vi "参数设置页.vi"() -> ()   [LabVIEW 2016, in "挥发酚.lvlib"]
uses:
  <vilib>/Plasmionique/MB Master/MB_Master/MB_Master.lvclass
  <vilib>/ptbypt/NI_PtbyPt.lvlib
panel:
  in  "维护模式":bool
  in  "标样核查自动补测":bool caption="通讯连接"
  in  "跨度核查自动补测":bool caption="通讯连接"
  in  "零点核查自动补测":bool caption="通讯连接"
  in  "标样核查标液偏差":dbl caption="标样核查标液偏差："
  in  "跨度核查标液偏差":dbl caption="跨度核查标液偏差："
  in  "零点核查标液偏差":dbl caption="零点核查标液偏差："
  out "error out":errorcluster
  out "数据刷新时间":string
  in  "通讯连接":bool
  out "MB table":enum32{"Serial", "TCP"}(tab)
  in  "请选择串口:":refnum<visa-resource-name>
  in  "IP":string="127.0.0.1"
  in  "PORT":string="1001"
  in  "通信方式选择":enum16{"串口", "TCP"}(ring)
  in  "刷新":bool
  in  "参数下拉列表":u16(ring)=1 items=["挥发酚"=1]
  in  "量程下拉列表":enum16{"低量程", "高量程"}(ring)
  out "量程下限":dbl caption="量程下限："
  out "量程上限":dbl caption="量程上限："
  out "检出限":dbl caption="检出限："
  out "曲线截距":dbl caption="曲线截距：" format="%#.6f"
  out "曲线斜率":dbl caption="曲线斜率：" format="%#.6f"
  out "二次多项式系数":dbl caption="二次多项式系数：" format="%#.6f"
  out "消解时长":dbl caption="消解时长："
  out "消解温度":dbl caption="消解温度："
  out "测量精度":dbl caption="测量精度："
  in  "标样核查标液浓度":dbl caption="标样核查标液浓度："
  in  "跨度核查标液浓度":dbl caption="跨度核查标液浓度："
  in  "零点核查标液浓度":dbl caption="零点核查标液浓度："
  in  "跨度值":dbl caption="跨度值："
  # "日质控设置"
  # "日质控自动补测设置"
  # "连接设置"
  # "±"
  # "%"
  # "%"
  # "关键参数"
  # "线性公式"
  # "mg/L"
  # "mg/L"
  # "mg/L"
  # "℃"
  # "min"
  # "mg/L"
  # "mg/L"
  # "mg/L"
  # "mg/L"
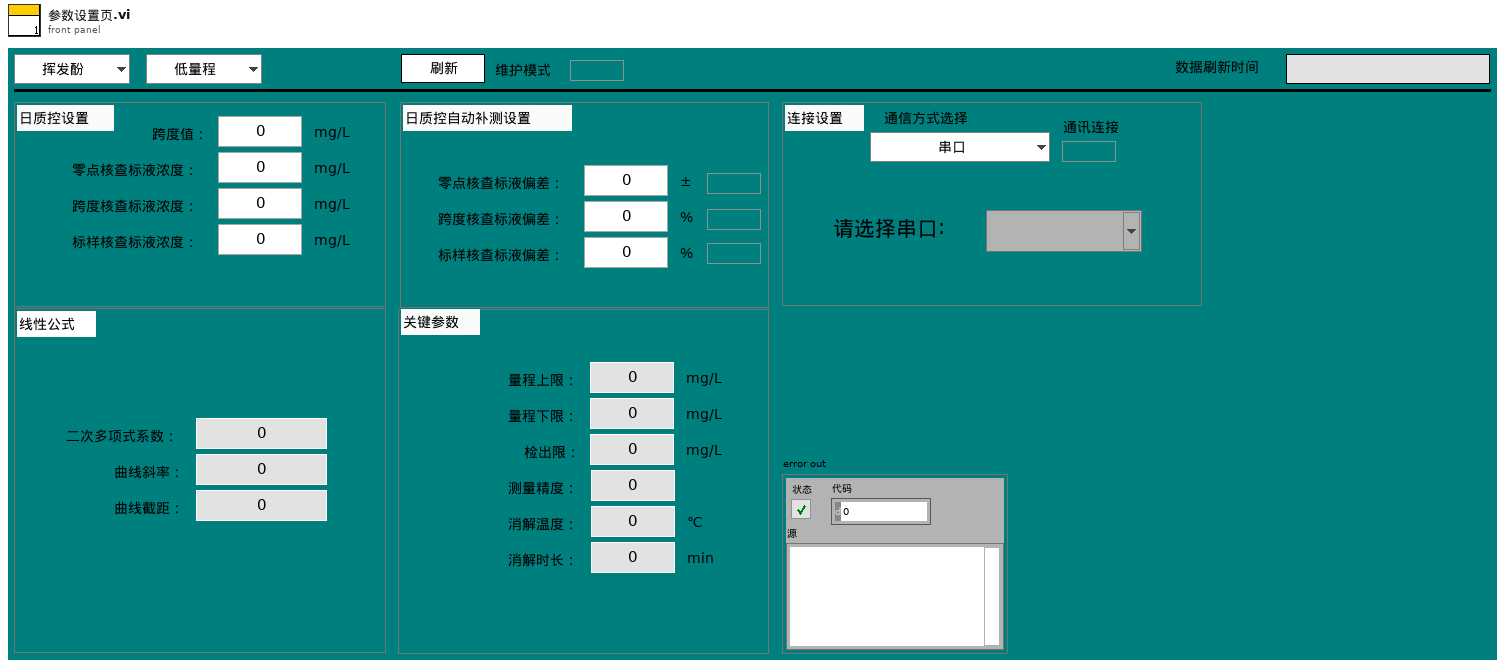
[diagram p1: front panel]
types:
  T1 = enum8{"Enabled", "Disabled", "Disabled and Grayed Out"}
  T2 = cluster{"跨度值":dbl, "零点标准液浓度":dbl, "跨度标准液浓度":dbl, "标准液标准浓度":dbl, "零点标准液偏差":dbl, "跨度标准液偏差":dbl, "标准液标准偏差":dbl}
  T3 = cluster{"测量量程":sgl, "测量检出限":sgl, "测量精度":sgl, "测量间隔":sgl, "消解温度":sgl, "消解时长":sgl, "三项式系数":sgl, "二次多项式系数":sgl, "曲线斜率":sgl, "曲线截距":sgl, "线性相关系数":sgl, "空白校准时间":timestamp, "标样校准时间":timestamp, "测量信号值":sgl, "稀释倍数":sgl, "量程系数":sgl}
  T4 = cluster{"测量精度":u16, "消解温度":u16, "消解时长":u16, "量程下限":sgl, "量程上限":sgl, "曲线斜率K":sgl, "曲线斜率B":sgl, "标定日期":timestamp, "标液1浓度":sgl, "标液1测量过程值":sgl, "标液2浓度":sgl, "标液2测量过程值":sgl, "标液3浓度":sgl, "标液3测量过程值":sgl, "标液4浓度":sgl, "标液4测量过程值":sgl, "标液5浓度":sgl, "标液5测量过程值":sgl, "线性相关系数":sgl, "试剂余量":u32, "测量滴定值或吸光度":sgl, "标样2校准时间":timestamp, "检出限值":sgl, "校准系数":sgl, "设备系列号":string, "显色温度":u16, "显色时间":u16, "试剂余量1":u16, "试剂余量2":u16, "试剂余量3":u16, "试剂余量4":u16, "试剂余量5":u16, "试剂余量6":u16, "试剂余量7":u16, "试剂余量8":u16, "试剂余量9":u16, "试剂余量10":u16, "当前量程低位":sgl, "当前量程高位":sgl}
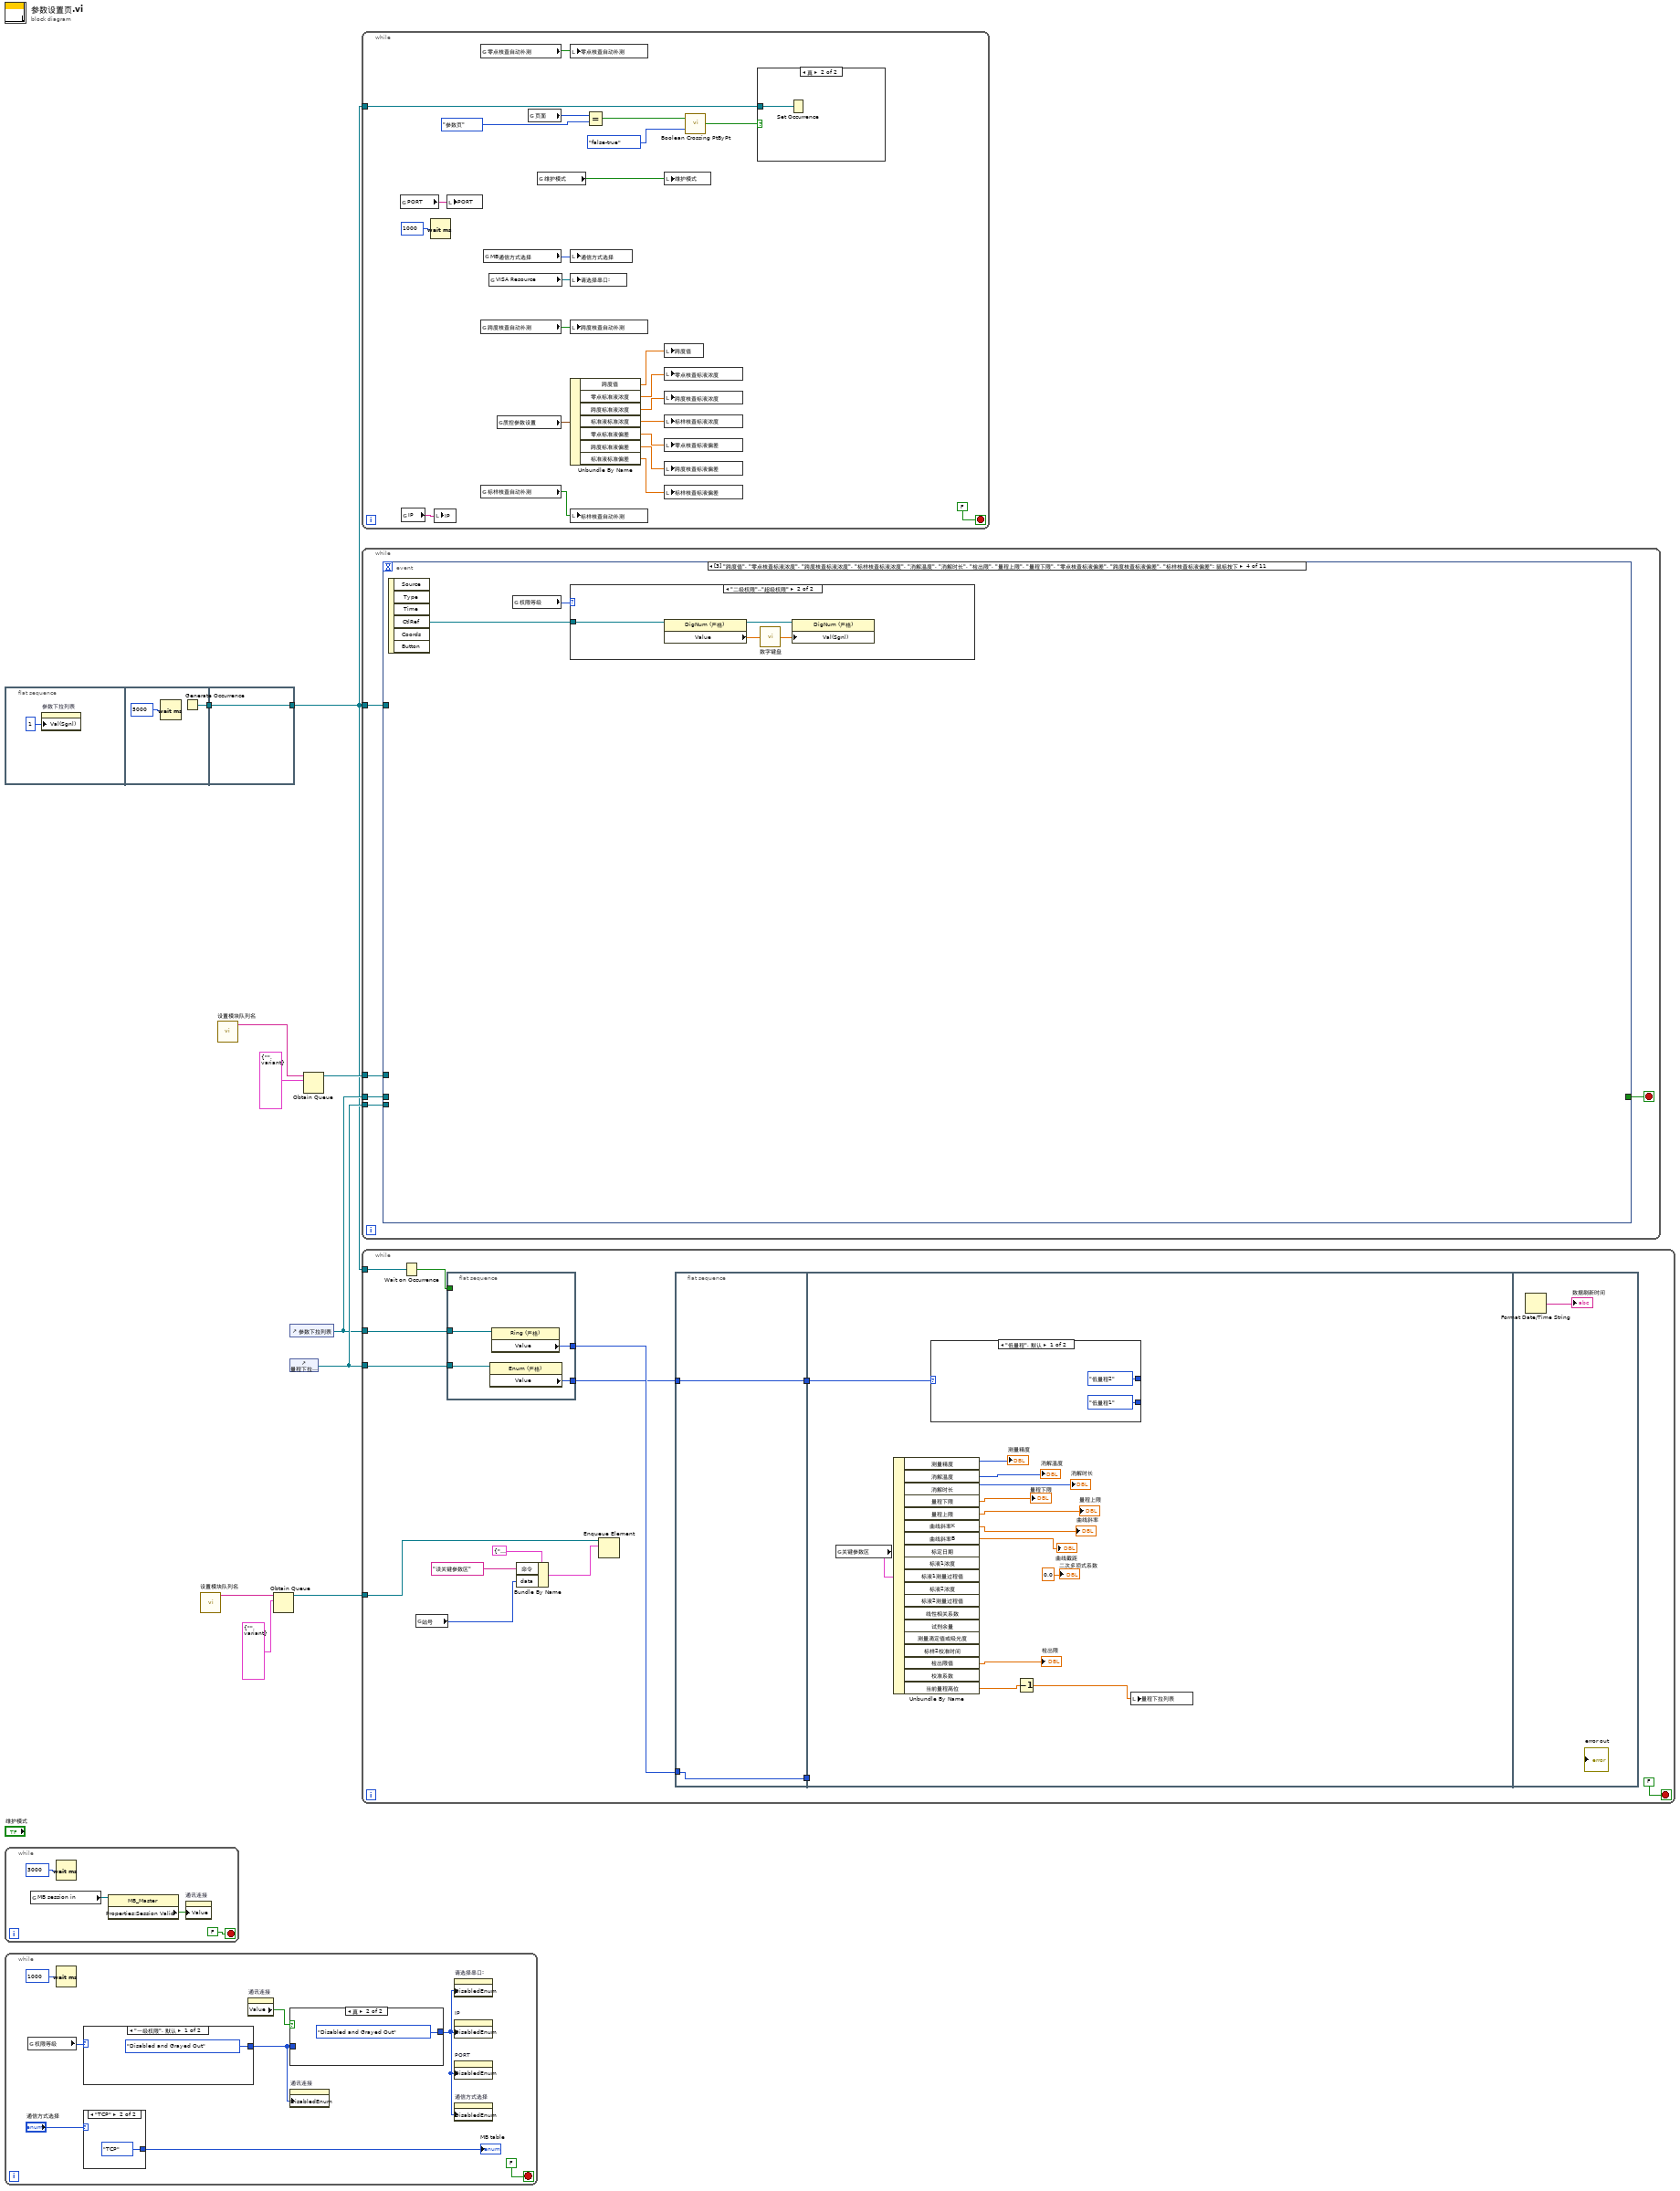
[diagram p0: block diagram]
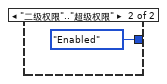
[diagram p3: hidden frame]
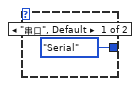
[diagram p4: hidden frame]
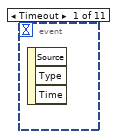
[diagram p6: hidden frame]
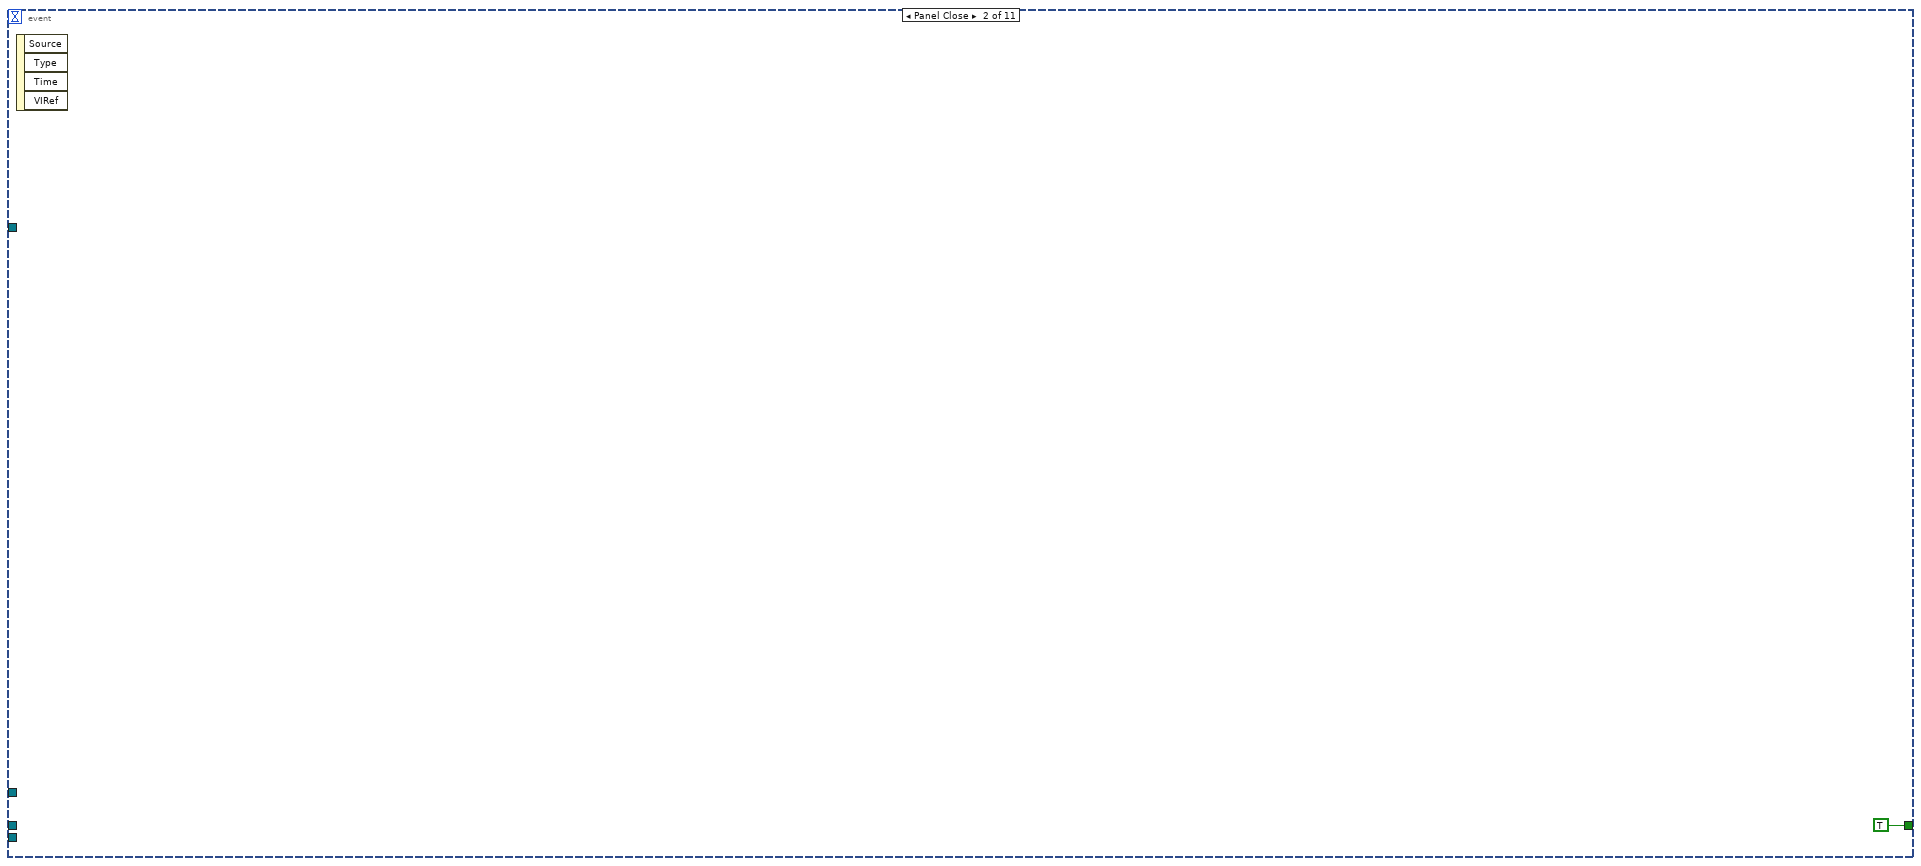
[diagram p7: hidden frame]
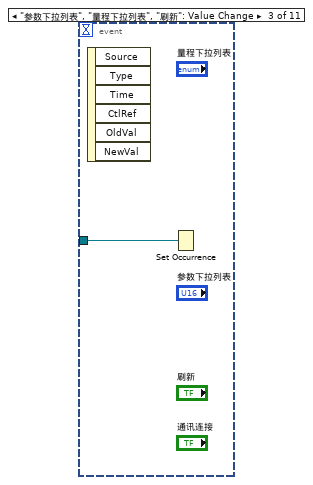
[diagram p8: hidden frame]
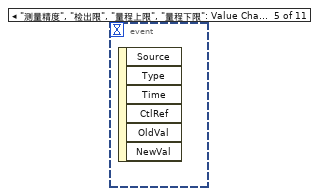
[diagram p10: hidden frame]
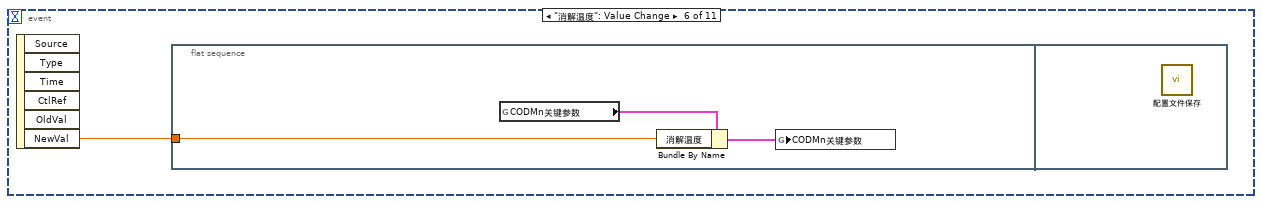
[diagram p11: hidden frame]
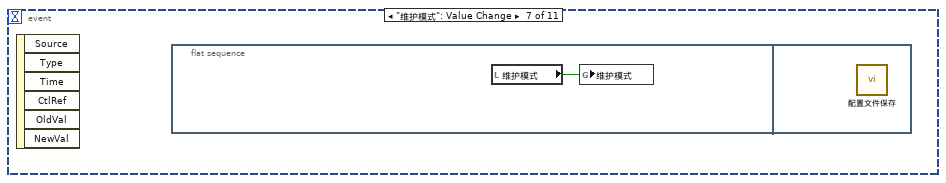
[diagram p12: hidden frame]
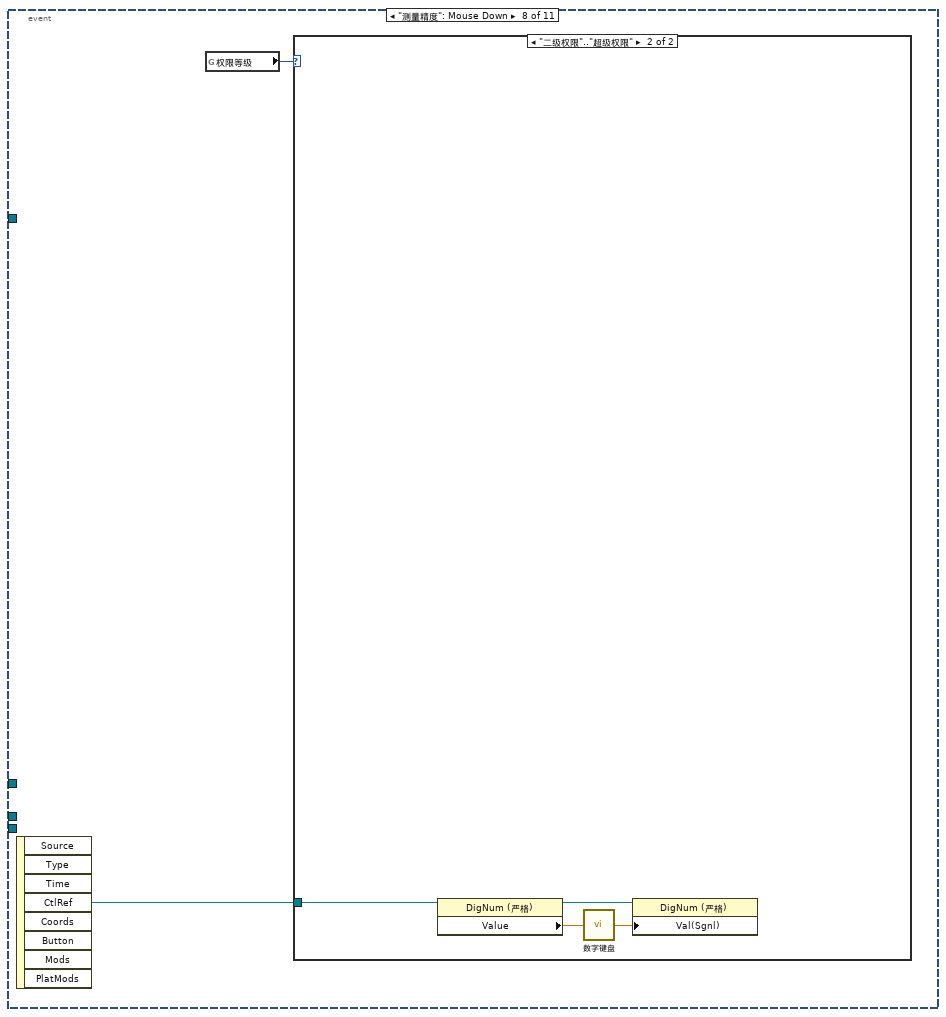
[diagram p13: hidden frame]
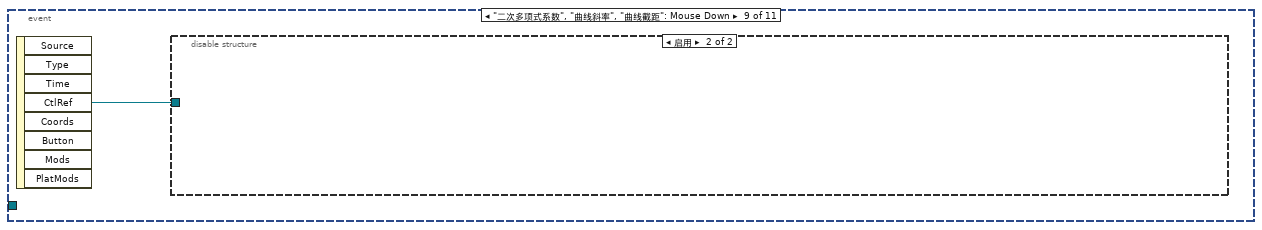
[diagram p15: hidden frame]
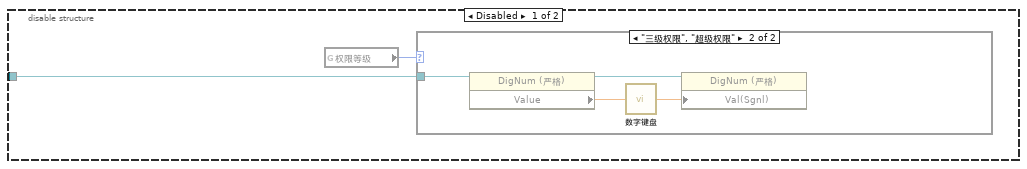
[diagram p16: hidden frame]
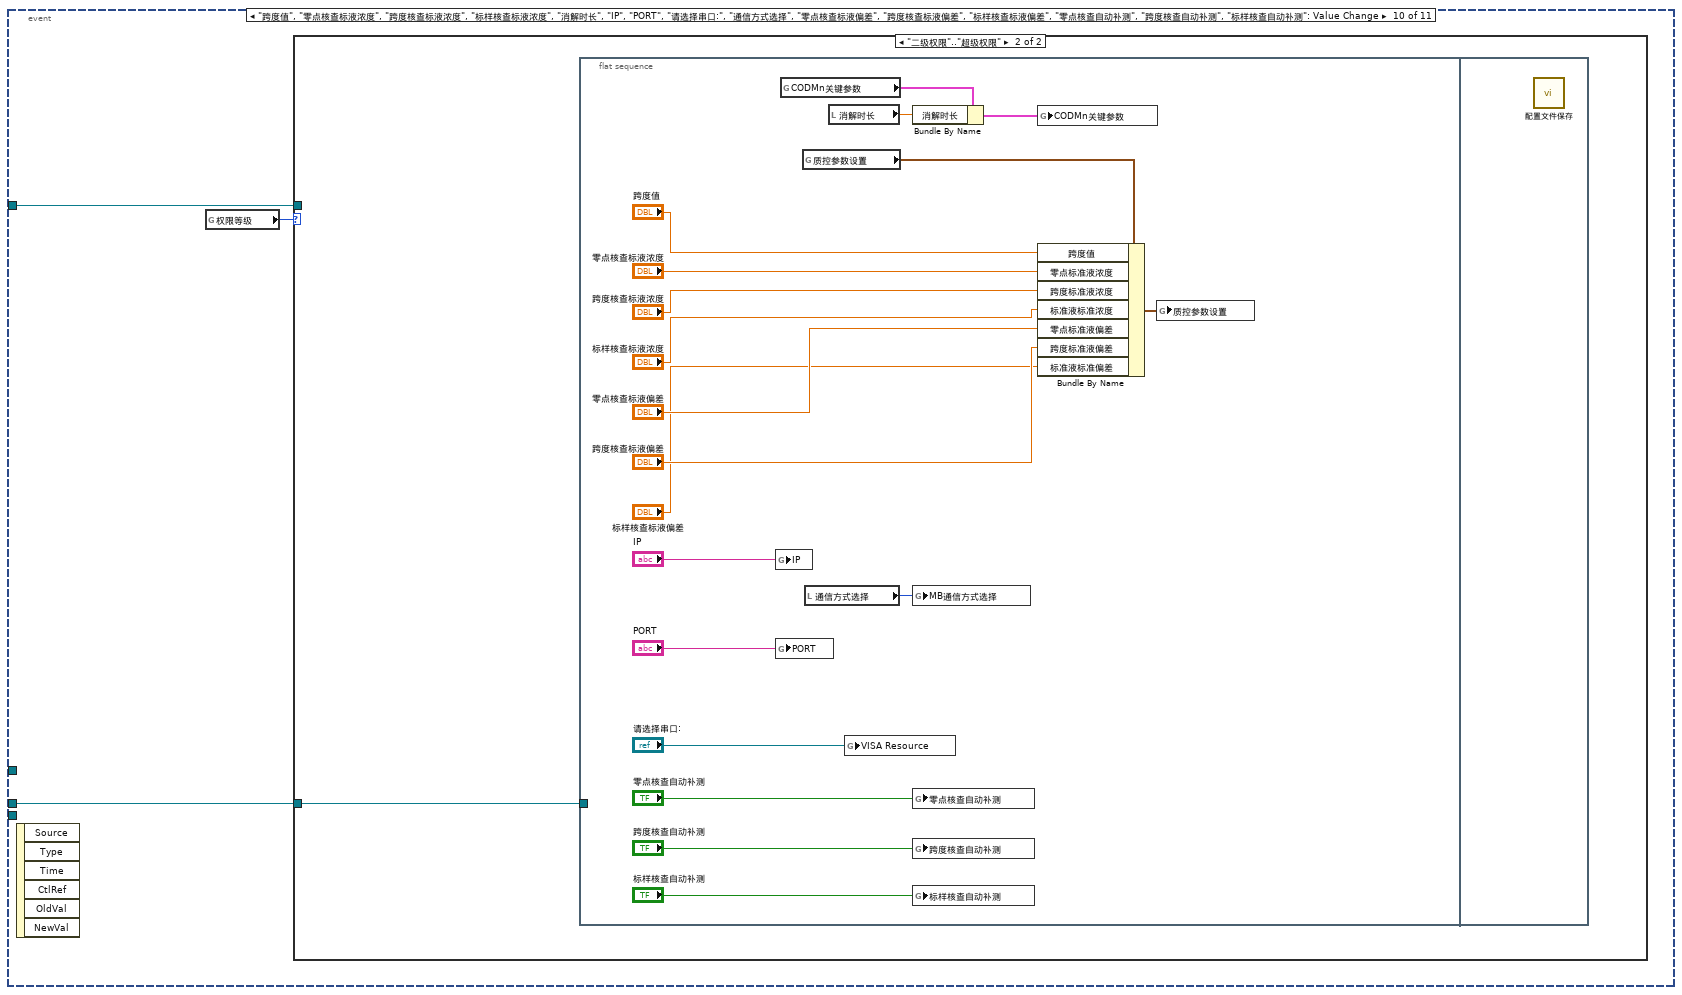
[diagram p18: hidden frame]
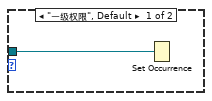
[diagram p19: hidden frame]
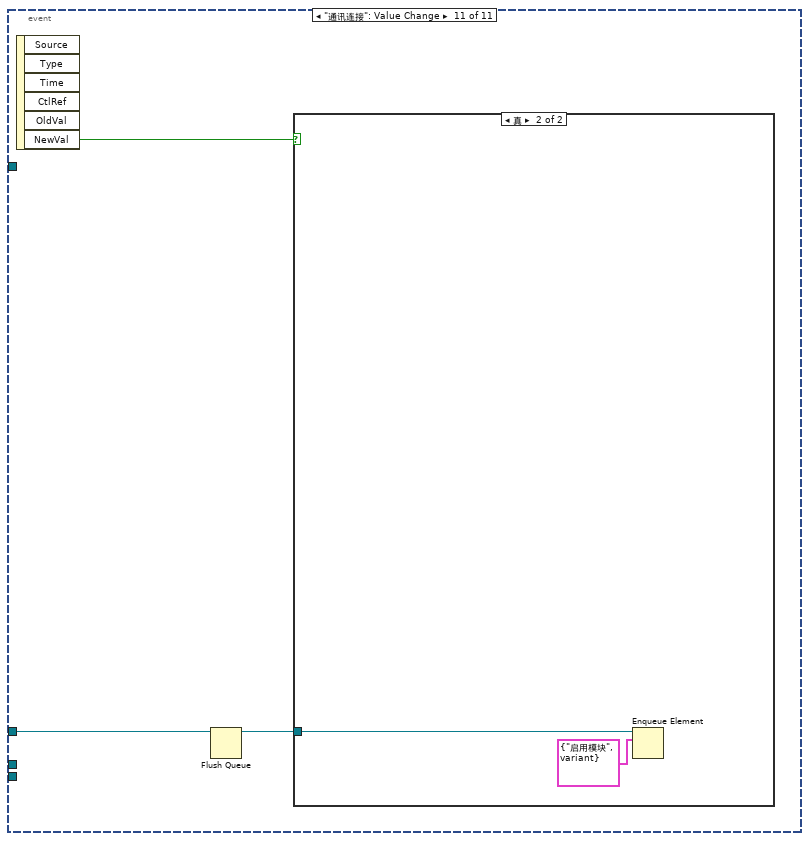
[diagram p20: hidden frame]
diagram:
  n1 = flat-sequence {
    tunnel: [w13] -> w10
    tunnel: [w14] -> w5
    tunnel: w10 -> [w14]
    frame #0 {
      n2 = property on="参数下拉列表" class="Ring (严格)"("Val(Sgnl)"=u16 1 ("值(信号)")) -> ()  [unwired: 2 in, 2 out]
    }
    frame #1 {
      n3 = Wait (ms)(milliseconds to wait=u32 5000 ("等待时间（毫秒）")) -> ()  [unwired: 1 out]
      n4 = Generate Occurrence() -> (w13:refnum<k4>)
    }
    frame #2 {
    }
  }
  n5 = while {
    stop <- FALSE stop-if-true
    n6 = global read "VAR挥发酚全局变量.vi" "MB session in"() -> (w17:refnum<class "MB_Master.lvclass">)
    n7 = Wait (ms)(milliseconds to wait=u32 3000 ("等待时间（毫秒）")) -> ()  [unwired: 1 out]
    n8 = property class="MB_Master"(reference=w17) -> ("Properties:Session Valid"=w16:bool)  [unwired: 1 in, 2 out]
    n9 = property on="通讯连接" class="Bool (严格)"("Value"=w16) -> ()  [unwired: 2 in, 2 out]
  }
  n10 = while {
    stop <- FALSE stop-if-true
    n11 = global read "VAR挥发酚全局变量.vi" "权限等级"() -> (w19:enum16{"一级权限", "二级权限", "三级权限", "超级权限"})
    n12 = Wait (ms)(milliseconds to wait=u32 1000 ("等待时间（毫秒）")) -> ()  [unwired: 1 out]
    n13 = case shown="\"一级权限\", 默认" w19 {
      tunnel: [T1."Disabled and Grayed Out" ("禁用") T1."Enabled" ("禁用")] -> w20
      frame "一级权限", Default {
      }
      frame "二级权限".."超级权限" {
      }
    }
    n14 = case shown="\"TCP\"" "通信方式选择" {
      tunnel: [enum32{"Serial", "TCP"}."Serial" ("MB table") enum32{"Serial", "TCP"}."TCP" ("MB table")] -> w22
      frame "串口", Default {
      }
      frame "TCP" {
      }
    }
    "MB table" <- w22
    n15 = property on="通讯连接" class="Bool (严格)"() -> ("Value"=w24:bool)  [unwired: 2 in, 2 out]
    n16 = case shown="真" w24 {
      tunnel: [w31 T1."Disabled and Grayed Out" ("禁用")] -> w23
      tunnel: w20 -> [w31 _]
      frame False {
      }
      frame True {
      }
    }
    n17 = property on="通讯连接" class="Bool (严格)"("DisabledEnum"=w20) -> ()  [unwired: 2 in, 2 out]
    n18 = property on="请选择串口:" class="VISAName"("DisabledEnum"=w23) -> ()  [unwired: 2 in, 2 out]
    n19 = property on="IP" class="Str"("DisabledEnum"=w23) -> ()  [unwired: 2 in, 2 out]
    n20 = property on="PORT" class="Str"("DisabledEnum"=w23) -> ()  [unwired: 2 in, 2 out]
    n21 = property on="通信方式选择" class="Enum (严格)"("DisabledEnum"=w23) -> ()  [unwired: 2 in, 2 out]
  }
  n22 = call "设置模块队列名.vi"() -> ("Msg"=w2:string)  [unwired: 11 in]
  n23 = call "设置模块队列名.vi"() -> ("Msg"=w4:string)  [unwired: 11 in]
  n24 = Obtain Queue(name (unnamed)=w2, element data type=cluster{"命令":string, "data":variant} {"命令"="", "data"=variant}) -> (queue out=w1:refnum<queue>)  [unwired: 3 in, 2 out]
  n25 = control-ref of="参数下拉列表"() -> (w6:refnum<vi>)
  n26 = control-ref of="量程下拉列表"() -> (w7:refnum<vi>)
  n27 = Obtain Queue(name (unnamed)=w4, element data type=cluster{"命令":string, "data":variant} {"命令"="", "data"=variant}) -> (queue out=w8:refnum<queue>)  [unwired: 3 in, 2 out]
  n28 = while {
    tunnel: w5 -> [w40]
    stop <- FALSE stop-if-true
    n29 = global read "挥发酚断电保存全局变量.vi" "PORT"() -> (w53:string)
    n30 = global read "挥发酚断电保存全局变量.vi" "IP"() -> (w52:string)
    n31 = Wait (ms)(milliseconds to wait=u32 1000 ("等待时间（毫秒）")) -> ()  [unwired: 1 out]
    n32 = local write "IP"(w52) -> ()
    n33 = local write "PORT"(w53) -> ()
    n34 = global read "挥发酚断电保存全局变量.vi" "零点核查自动补测"() -> (w35:bool)
    n35 = global read "挥发酚断电保存全局变量.vi" "跨度核查自动补测"() -> (w34:bool)
    n36 = global read "挥发酚断电保存全局变量.vi" "标样核查自动补测"() -> (w39:bool)
    n37 = global read "挥发酚断电保存全局变量.vi" "MB通信方式选择"() -> (w51:enum16{"串口", "TCP"})
    n38 = global read "挥发酚断电保存全局变量.vi" "VISA Resource"() -> (w54:refnum<visa-resource-name>)
    n39 = global read "挥发酚断电保存全局变量.vi" "质控参数设置"() -> (w46:T2)
    n40 = global read "VAR挥发酚全局变量.vi" "页面"() -> (w45:enum16{"主页", "参数页", "校准页"})
    n41 = global read "挥发酚断电保存全局变量.vi" "维护模式"() -> (w33:bool)
    n42 = local write "零点核查自动补测"(w35) -> ()
    n43 = local write "通信方式选择"(w51) -> ()
    n44 = local write "请选择串口:"(w54) -> ()
    n45 = local write "跨度核查自动补测"(w34) -> ()
    n46 = Unbundle By Name(w46) -> ("跨度值"=w47:dbl, "零点标准液浓度"=w48:dbl, "跨度标准液浓度"=w49:dbl, "标准液标准浓度"=w50:dbl, "零点标准液偏差"=w38:dbl, "跨度标准液偏差"=w37:dbl, "标准液标准偏差"=w36:dbl)
    n47 = local write "标样核查自动补测"(w39) -> ()
    n48 = Equal?(x=w45, y=enum16{"主页", "参数页", "校准页"}."参数页") -> (x = y?=w43:bool)
    n49 = local write "维护模式"(w33) -> ()
    n50 = local write "跨度值"(w47) -> ()
    n51 = local write "零点核查标液浓度"(w48) -> ()
    n52 = local write "跨度核查标液浓度"(w49) -> ()
    n53 = local write "标样核查标液浓度"(w50) -> ()
    n54 = local write "零点核查标液偏差"(w38) -> ()
    n55 = local write "跨度核查标液偏差"(w37) -> ()
    n56 = local write "标样核查标液偏差"(w36) -> ()
    n57 = call <vilib>:"Boolean Crossing PtByPt.vi"("direction"=enum16{"either", "false-true", "true-false"}."false-true", "input"=w43) -> ("crossing"=w41:bool)  [unwired: 1 in]
    n58 = case shown="真" w41 {
      tunnel: w40 -> [_ w57]
      frame False {
      }
      frame True {
        n59 = Set Occurrence(w57) -> ()
      }
    }
  }
  n60 = while {
    tunnel: w5 -> [w61]
    tunnel: w6 -> [w60]
    tunnel: w8 -> [w59]
    tunnel: w7 -> [w58]
    stop <- w62 stop-if-true
    n61 = event shown="[3] \"跨度值\", \"零点核查标液浓度\", \"跨度核查标液浓度\", \"标样核查标液浓度\", \"消解温度\", \"消解时长\", \"检出限\", \"量程上限\", \"量程下限\", \"零点核查标液偏差\", \"跨度核查标液偏差\", \"标样核查标液偏差\": 鼠标按下" {
      selector: _ -> [_ _ _ _ _ _ _ _ _ _ _]
      dyn-events: _ -> [_ _ _ _ _ _ _ _ _ _ _]
      timeout: _ -> [_ _ _ _ _ _ _ _ _ _ _]
      tunnel: [_ TRUE _ _ _ _ _ _ _ _ _] -> w62
      tunnel: w61 -> [_ _ w64 _ _ _ _ _ _ w89 _]
      tunnel: w60 -> [_ _ _ _ _ _ _ _ _ w91 _]
      tunnel: w59 -> [_ _ _ _ _ _ _ _ _ _ w114]
      tunnel: w58 -> [_ _ _ _ _ _ _ _ _ _ _]
      event Timeout {
        n62 = event-data() -> ()  [unwired: 1 in, 3 out]
      }
      event Panel Close {
        n63 = event-data() -> ()  [unwired: 1 in, 4 out]
      }
      event "参数下拉列表", "量程下拉列表", "刷新": Value Change {
        n64 = event-data() -> ()  [unwired: 1 in, 6 out]
        n65 = Set Occurrence(w64) -> ()
      }
      event "跨度值", "零点核查标液浓度", "跨度核查标液浓度", "标样核查标液浓度", "消解温度", "消解时长", "检出限", "量程上限", "量程下限", "零点核查标液偏差", "跨度核查标液偏差", "标样核查标液偏差": Mouse Down {
        n66 = event-data() -> ("CtlRef"=w66:refnum<vi>)  [unwired: 1 in, 5 out]
        n67 = global read "VAR挥发酚全局变量.vi" "权限等级"() -> (w65:enum16{"一级权限", "二级权限", "三级权限", "超级权限"})
        n68 = case shown="\"二级权限\"..\"超级权限\"" w65 {
          tunnel: w66 -> [_ w70]
          frame "一级权限", Default {
          }
          frame "二级权限".."超级权限" {
            n69 = property class="DigNum (严格)"(reference=w70) -> (reference out=w68:refnum<vi>, "Value"=w69:dbl)  [unwired: 1 in, 1 out]
            n70 = call "数字键盘.vi"("OldNumber"=w69) -> ("NewNumber"=w67:dbl)
            n71 = property class="DigNum (严格)"(reference=w68, "Val(Sgnl)"=w67) -> ()  [unwired: 1 in, 2 out]
          }
        }
      }
      event "测量精度", "检出限", "量程上限", "量程下限": Value Change {
        n72 = event-data() -> ()  [unwired: 1 in, 6 out]
      }
      event "消解温度": Value Change {
        n73 = event-data() -> ("NewVal"=w71:dbl)  [unwired: 1 in, 5 out]
        n74 = flat-sequence {
          tunnel: w71 -> [w74]
          frame #0 {
            n75 = global read "挥发酚断电保存全局变量.vi" "CODMn关键参数"() -> (w72:T3)
            n76 = Bundle By Name(cluster=w72, "消解温度"=w74) -> (w73:T3)
            n77 = global write "挥发酚断电保存全局变量.vi" "CODMn关键参数"(w73) -> ()
          }
          frame #1 {
            n78 = call "配置文件保存.vi"() -> ()  [unwired: 12 in]
          }
        }
      }
      event "维护模式": Value Change {
        n79 = event-data() -> ()  [unwired: 1 in, 6 out]
        n80 = flat-sequence {
          frame #0 {
            n81 = local read "维护模式"() -> (w75:bool)
            n82 = global write "挥发酚断电保存全局变量.vi" "维护模式"(w75) -> ()
          }
          frame #1 {
            n83 = call "配置文件保存.vi"() -> ()  [unwired: 12 in]
          }
        }
      }
      event "测量精度": Mouse Down {
        n84 = event-data() -> ("CtlRef"=w77:refnum<vi>)  [unwired: 1 in, 7 out]
        n85 = global read "VAR挥发酚全局变量.vi" "权限等级"() -> (w76:enum16{"一级权限", "二级权限", "三级权限", "超级权限"})
        n86 = case shown="\"二级权限\"..\"超级权限\"" w76 {
          tunnel: w77 -> [_ w81]
          frame "一级权限", Default {
          }
          frame "二级权限".."超级权限" {
            n87 = property class="DigNum (严格)"(reference=w81) -> (reference out=w79:refnum<vi>, "Value"=w80:dbl)  [unwired: 1 in, 1 out]
            n88 = call "数字键盘.vi"("OldNumber"=w80) -> ("NewNumber"=w78:dbl)
            n89 = property class="DigNum (严格)"(reference=w79, "Val(Sgnl)"=w78) -> ()  [unwired: 1 in, 2 out]
          }
        }
      }
      event "二次多项式系数", "曲线斜率", "曲线截距": Mouse Down {
        n90 = event-data() -> ("CtlRef"=w82:refnum<vi>)  [unwired: 1 in, 7 out]
        n91 = disable-structure shown="启用" {
          disable-tunnel: w82 -> [w84 _]
          frame Disabled {
            n92 = global read "VAR挥发酚全局变量.vi" "权限等级"() -> (w83:enum16{"一级权限", "二级权限", "三级权限", "超级权限"})
            n93 = case shown="\"三级权限\", \"超级权限\"" w83 {
              tunnel: w84 -> [_ w88]
              frame "一级权限", Default {
              }
              frame "三级权限", "超级权限" {
                n94 = property class="DigNum (严格)"(reference=w88) -> (reference out=w86:refnum<vi>, "Value"=w87:dbl)  [unwired: 1 in, 1 out]
                n95 = call "数字键盘.vi"("OldNumber"=w87) -> ("NewNumber"=w85:dbl)
                n96 = property class="DigNum (严格)"(reference=w86, "Val(Sgnl)"=w85) -> ()  [unwired: 1 in, 2 out]
              }
            }
          }
          frame Enabled {
          }
        }
      }
      event "跨度值", "零点核查标液浓度", "跨度核查标液浓度", "标样核查标液浓度", "消解时长", "IP", "PORT", "请选择串口:", "通信方式选择", "零点核查标液偏差", "跨度核查标液偏差", "标样核查标液偏差", "零点核查自动补测", "跨度核查自动补测", "标样核查自动补测": Value Change {
        n97 = event-data() -> ()  [unwired: 1 in, 6 out]
        n98 = global read "VAR挥发酚全局变量.vi" "权限等级"() -> (w90:enum16{"一级权限", "二级权限", "三级权限", "超级权限"})
        n99 = case shown="\"二级权限\"..\"超级权限\"" w90 {
          tunnel: w91 -> [_ w93]
          tunnel: w89 -> [w92 _]
          frame "一级权限", Default {
            n100 = Set Occurrence(w92) -> ()
          }
          frame "二级权限".."超级权限" {
            n101 = flat-sequence {
              tunnel: w93 -> [_]
              frame #0 {
                n102 = global write "挥发酚断电保存全局变量.vi" "IP"("IP") -> ()
                n103 = global write "挥发酚断电保存全局变量.vi" "PORT"("PORT") -> ()
                n104 = global read "挥发酚断电保存全局变量.vi" "CODMn关键参数"() -> (w101:T3)
                n105 = global read "挥发酚断电保存全局变量.vi" "质控参数设置"() -> (w108:T2)
                n106 = local read "通信方式选择"() -> (w104:enum16{"串口", "TCP"})
                n107 = local read "消解时长"() -> (w103:dbl)
                n108 = global write "挥发酚断电保存全局变量.vi" "VISA Resource"("请选择串口:") -> ()
                n109 = Bundle By Name(cluster=w101, "消解时长"=w103) -> (w100:T3)
                n110 = global write "挥发酚断电保存全局变量.vi" "MB通信方式选择"(w104) -> ()
                n111 = global write "挥发酚断电保存全局变量.vi" "零点核查自动补测"("零点核查自动补测") -> ()
                n112 = global write "挥发酚断电保存全局变量.vi" "跨度核查自动补测"("跨度核查自动补测") -> ()
                n113 = global write "挥发酚断电保存全局变量.vi" "标样核查自动补测"("标样核查自动补测") -> ()
                n114 = global write "挥发酚断电保存全局变量.vi" "CODMn关键参数"(w100) -> ()
                n115 = Bundle By Name(cluster=w108, "跨度值"="跨度值", "零点标准液浓度"="零点核查标液浓度", "跨度标准液浓度"="跨度核查标液浓度", "标准液标准浓度"="标样核查标液浓度", "零点标准液偏差"="零点核查标液偏差", "跨度标准液偏差"="跨度核查标液偏差", "标准液标准偏差"="标样核查标液偏差") -> (w102:T2)
                n116 = global write "挥发酚断电保存全局变量.vi" "质控参数设置"(w102) -> ()
              }
              frame #1 {
                n117 = call "配置文件保存.vi"() -> ()  [unwired: 12 in]
              }
            }
          }
        }
      }
      event "通讯连接": Value Change {
        n118 = event-data() -> ("NewVal"=w113:bool)  [unwired: 1 in, 5 out]
        n119 = Flush Queue(queue=w114) -> (queue out=w115:refnum<queue>)  [unwired: 1 in, 2 out]
        n120 = case shown="真" w113 {
          tunnel: w115 -> [w116 w118]
          frame False {
            n121 = Enqueue Element(queue=w116, element=cluster{"命令":string, "data":variant} {"命令"="停用模块", "data"=variant} ("元素")) -> ()  [unwired: 2 in, 3 out]
          }
          frame True {
            n122 = Enqueue Element(queue=w118, element=cluster{"命令":string, "data":variant} {"命令"="启用模块", "data"=variant} ("元素")) -> ()  [unwired: 2 in, 3 out]
          }
        }
      }
    }
  }
  n123 = while {
    tunnel: w6 -> [w132]
    tunnel: w7 -> [w131]
    tunnel: w5 -> [w130]
    tunnel: w1 -> [w121]
    stop <- FALSE stop-if-true
    n124 = Wait on Occurrence(2:w130) -> (0:w126:bool)  [unwired: 2 in]
    n125 = global read "挥发酚断电保存全局变量.vi" "站号"() -> (w120:u16)
    n126 = flat-sequence {
      tunnel: w132 -> [w137]
      tunnel: w131 -> [w136]
      tunnel: [w135] -> w128
      tunnel: [w134] -> w127
      tunnel: w126 -> [_]
      frame #0 {
        n127 = property class="Enum (严格)"(reference=w136) -> ("Value"=w134:enum16{"低量程", "高量程"})  [unwired: 1 in, 2 out]
        n128 = property class="Ring (严格)"(reference=w137) -> ("Value"=w135:u16)  [unwired: 1 in, 2 out]
      }
    }
    n129 = Bundle By Name(cluster=cluster{"命令":string, "data":variant} {"命令"="", "data"=variant} ("元素"), "命令"="读关键参数区", "data"=w120) -> (w123:cluster{"命令":string, "data":variant})
    n130 = Enqueue Element(queue=w121, element=w123) -> ()  [unwired: 2 in, 3 out]
    n131 = flat-sequence {
      tunnel: [w139] -> w129
      tunnel: w128 -> [w138]
      tunnel: w127 -> [w139]
      tunnel: [w138] -> w125
      tunnel: w129 -> [w152]
      tunnel: w125 -> [_]
      frame #0 {
      }
      frame #1 {
        n132 = global read "VAR挥发酚全局变量.vi" "关键参数区"() -> (w151:T4)
        n133 = Unbundle By Name(w151) -> ("测量精度"=→"测量精度":u16, "消解温度"=→"消解温度":u16, "消解时长"=→"消解时长":u16, "量程下限"=→"量程下限":sgl, "量程上限"=→"量程上限":sgl, "曲线斜率K"=→"曲线斜率":sgl, "曲线斜率B"=→"曲线截距":sgl, "检出限值"=→"检出限":sgl, "当前量程高位"=w141:sgl)  [unwired: 10 out]
        n134 = case shown="\"低量程\", 默认" w152 {
          tunnel: [enum16{"低量程1", "低量程2", "高量程1", "高量程2"}."低量程1" ("量程") enum16{"低量程1", "低量程2", "高量程1", "高量程2"}."高量程1" ("量程")] -> _
          tunnel: [enum16{"低量程1", "低量程2", "高量程1", "高量程2"}."低量程2" ("量程") enum16{"低量程1", "低量程2", "高量程1", "高量程2"}."高量程2" ("量程")] -> _
          frame "低量程", Default {
          }
          frame "高量程" {
          }
        }
        n135 = Decrement(x=w141) -> (x-1=w140:sgl)
        n136 = local write "量程下拉列表"(w140) -> ()
        "二次多项式系数" <- 0.0 ("二次多项式系数")
      }
      frame #2 {
        n137 = Format Date/Time String() -> (date/time string=→"数据刷新时间":string)  [unwired: 3 in]
      }
    }
  }
